vi "add_fit_to_plot.vi"(9 "fit_Best_Fit_results":dbl[](array[numeric]), 10 "x-Array":dbl[](array[numeric]), 11 "XY Graph in":refnum<vi>) -> ()   [LabVIEW 2017]
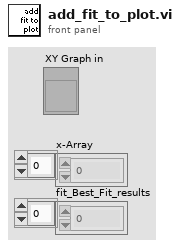
[diagram p1: front panel]
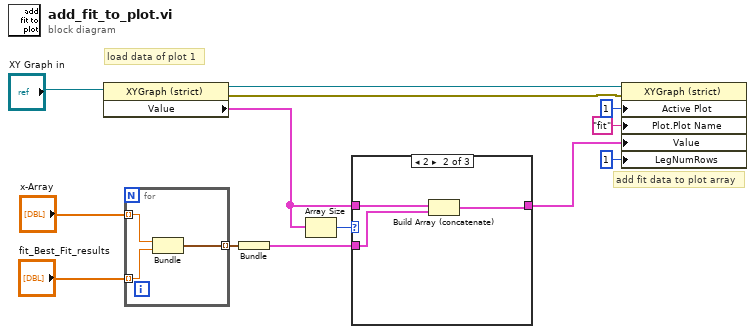
[diagram p0: block diagram]
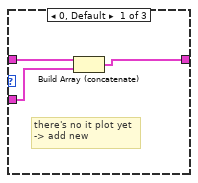
[diagram p2: hidden frame]
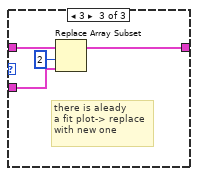
[diagram p3: hidden frame]
diagram:
  # "add fit data to plot array"
  # "load data of plot 1"
  n1 = property class="XYGraph (strict)"(reference="XY Graph in") -> (reference out=w9:refnum<vi>, error out=w8:errorcluster, "Value"=w1:cluster{cluster{"x":dbl, "y":dbl}[]}[])  [unwired: 1 in]
  n2 = for {
    tunnel: "x-Array" -> [w16] mode=indexing
    tunnel: "fit_Best_Fit_results" -> [w15] mode=indexing
    tunnel: [w14] -> w6 mode=indexing
    n3 = Bundle("X"=w16, "Numeric"=w15) -> (w14:cluster{"X":dbl, "Numeric":dbl})  [unwired: 1 in]
  }
  n4 = Bundle(w6) -> (w4:cluster{cluster{"X":dbl, "Numeric":dbl}[]})  [unwired: 1 in]
  n5 = Array Size(array=w1) -> (size(s)=w2:i32)
  n6 = case shown="2" w2 {
    tunnel: w1 -> [w19 w22 w26]
    tunnel: w4 -> [w18 w21 w25]
    tunnel: [w17 w20 w23] -> w3
    frame 0, Default {
      # "there's no it plot yet\n-> add new"
      n7 = Build Array (concatenate)(w19, w18) -> (w17:cluster{cluster{"X":dbl, "Numeric":dbl}[]}[])
    }
    frame 2 {
      n8 = Build Array (concatenate)(w22, w21) -> (w20:cluster{cluster{"X":dbl, "Numeric":dbl}[]}[])
    }
    frame 3 {
      # "there is aleady\na fit plot-> replace\nwith new one"
      n9 = Replace Array Subset(array=w26, new element=w25, index=2) -> (w23:cluster{cluster{"x":dbl, "y":dbl}[]}[])
    }
  }
  n10 = property class="XYGraph (strict)"(reference=w9, error in=w8, "Active Plot"=u32 1, "Plot.Plot Name"="fit", "Value"=w3, "LegNumRows"=u32 1 ("Legend:Number of Rows")) -> ()  [unwired: 2 out]
